vi "Test Deserialize Source Path.vi"(8 "error in (no error)":errorcluster) -> (0 "error out":errorcluster)   [LabVIEW 2020]
uses:
  <vilib>/addons/_JKI Toolkits/Caraya/classes/Assert/Assert True.vi
  <vilib>/regexp/Match Regular Expression.xnode
  <vilib>/addons/_JKI Toolkits/Caraya/classes/Test/Test.lvclass
  src/JKI JSON Serialization.lvlib
  <vilib>/addons/_JKI Toolkits/Caraya/classes/Assert/Assert.lvclass
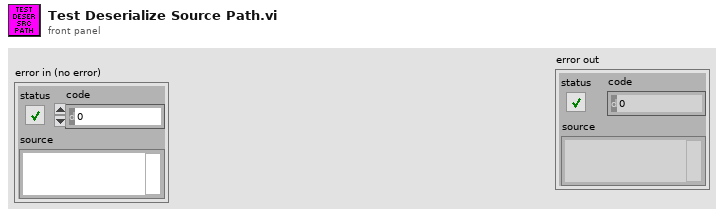
[diagram p1: front panel]
types:
  T1 = cluster{"test label":string, "source path":string, "input json":string, "error match":string}[]
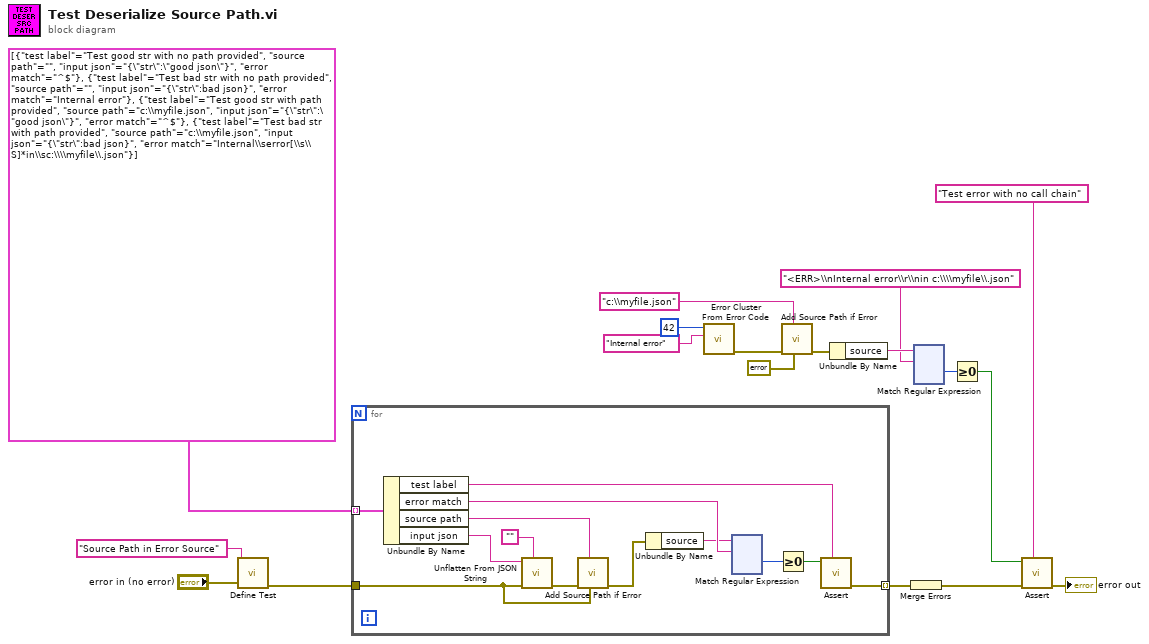
[diagram p0: block diagram]
diagram:
  n1 = call <vilib>:"Define Test.vi"("error in (no error)"="error in (no error)", "Label (VI Title)"="Source Path in Error Source") -> ("error out"=w15:errorcluster)  [unwired: 8 in, 1 out]
  n2 = for {
    tunnel: w15 -> [w20]
    tunnel: [w31] -> w16 mode=indexing
    tunnel: T1 [{"test label"="Test good str with no path provided", "source path"="", "input json"="{\"str\":\"good json\"}", "error match"="^$"}, {"test label"="Test bad str with no path provided", "source path"="", "input json"="{\"str\":bad json}", "error match"="Internal error"}, {"test label"="Test good str with path provided", "source path"="c:\\myfile.json", "input json"="{\"str\":\"good json\"}", "error match"="^$"}, {"test label"="Test bad str with path provided", "source path"="c:\\myfile.json", "input json"="{\"str\":bad json}", "error match"="Internal\\serror[\\s\\S]*in\\sc:\\\\myfile\\.json"}] -> [w30] mode=indexing
    n3 = Unbundle By Name(w30) -> ("test label"=w29:string, "error match"=w26:string, "source path"=w21:string, "input json"=w28:string)
    n4 = call "Unflatten From JSON String.vi"("Type and Defaults"="", "error in (no error)"=w20, "JSON String"=w28) -> ("error out"=w22:errorcluster)  [unwired: 7 in, 1 out]
    n5 = call "Add Source Path if Error.vi"("Upstream Error"=w20, "Source Path or URL"=w21, "error in (no error)"=w22) -> ("error out"=w19:errorcluster)  [unwired: 8 in]
    n6 = Unbundle By Name(w19) -> ("source"=w23:string)
    n7 = xnode ("Match Regular Expression")("input string"=w23, "regular expression"=w26) -> ("offset past match"=w25:i32)  [unwired: 4 in, 4 out]
    n8 = Greater Or Equal To 0?(x=w25) -> (x >= 0?=w24:bool)
    n9 = call-poly <vilib>:"Assert.vi"("Label"=w29, "True?"=w24) -> ("error out"=w31:errorcluster)  [unwired: 8 in, 1 out]
  }
  n10 = call <vilib>:"Error Cluster From Error Code.vi"("error message (\"\")"="Internal error" ("error message (\"\")"), "error code (0)"=42) -> ("error out"=w10:errorcluster)  [unwired: 7 in]
  n11 = call "Add Source Path if Error.vi"("Upstream Error"=errorcluster {"status"=FALSE, "code"=0, "source"=""}, "Source Path or URL"="c:\\myfile.json" ("source path"), "error in (no error)"=w10) -> ("error out"=w7:errorcluster)  [unwired: 8 in]
  n12 = Unbundle By Name(w7) -> ("source"=w5:string)
  n13 = Merge Errors(w16) -> (w13:errorcluster)
  n14 = xnode ("Match Regular Expression")("input string"=w5, "regular expression"="<ERR>\\nInternal error\\r\\nin c:\\\\myfile\\.json" ("Label")) -> ("offset past match"=w6:i32)  [unwired: 4 in, 4 out]
  n15 = Greater Or Equal To 0?(x=w6) -> (x >= 0?=w4:bool)
  n16 = call-poly <vilib>:"Assert.vi"("Label"="Test error with no call chain", "error in (no error)"=w13, "True?"=w4) -> ("error out"=→"error out":errorcluster)  [unwired: 7 in, 1 out]
